vi "VFH-save_R140.vi"(7 "file path (use dialog)":path, 8 "error in (no error)":errorcluster, 10 "input":T1) -> (0 "error out":errorcluster)   [LabVIEW 2020, in "VFH-VNA_File_Handler.lvlib"]
uses:
  VFH-VNA_File_Handler.lvlib
  VFH-file_cluster-R140.ctl
  <vilib>/Utility/file.llb/Write Delimited Spreadsheet (DBL).vi
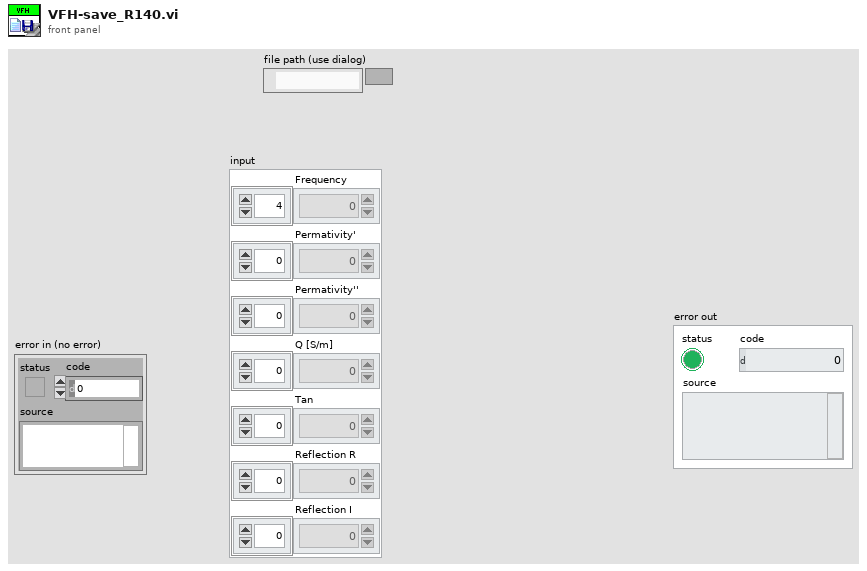
[diagram p1: front panel]
types:
  T1 = typedef "VFH-VNA_File_Handler.lvlib/VFH-file_cluster-R140.ctl" = cluster{"Frequency":dbl[], "Permativity'":dbl[], "Permativity''":dbl[], "Q [S/m]":dbl[], "Tan":dbl[], "Reflection R":dbl[], "Reflection I":dbl[]}
  T2 = enum16{"open", "replace", "create", "open or create", "replace or create", "replace or create with confirmation"}
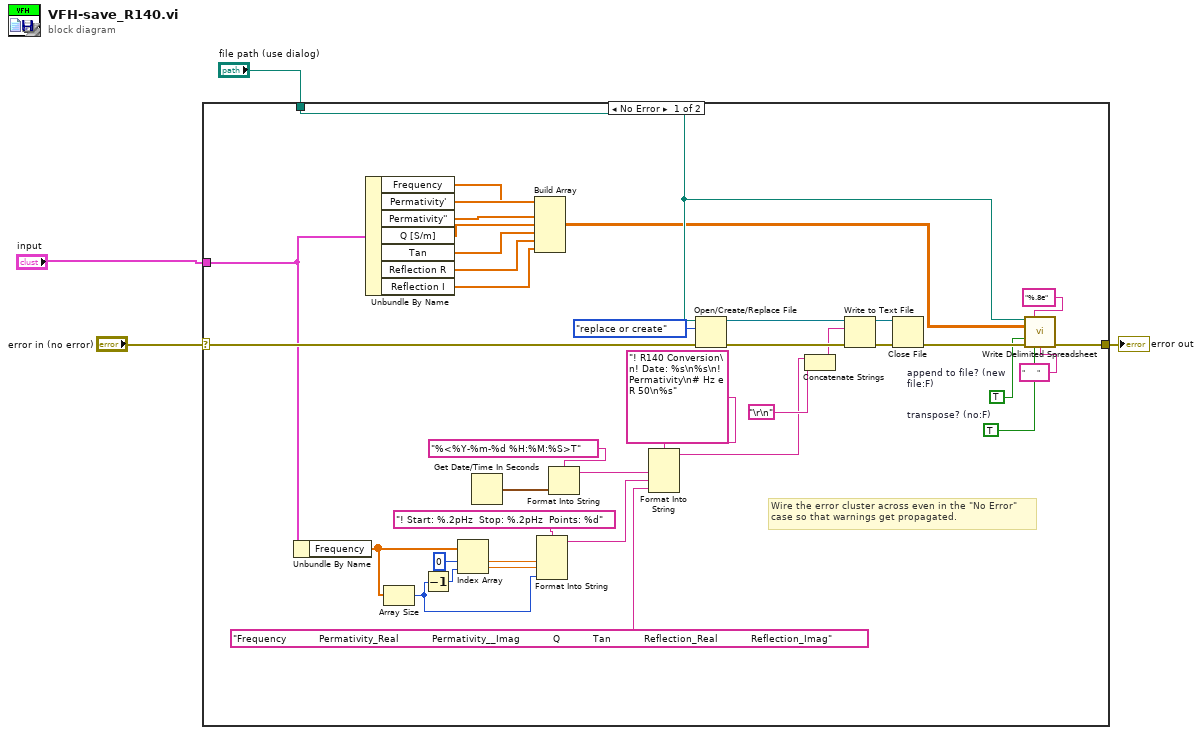
[diagram p0: block diagram]
diagram:
  n1 = case shown="No Error" "error in (no error)" {
    selector: "error in (no error)" -> [w13 w43]
    tunnel: [w5 w43] -> w1
    tunnel: "input" -> [w6 _]
    tunnel: "file path (use dialog)" -> [w22 _]
    frame No Error {
      w24 = TRUE  # append to file? (new file:F)
      w26 = TRUE  # transpose? (no:F)
      # "Wire the error cluster across even in the \"No Error\"\ncase so that warnings get propagated."
      n2 = Unbundle By Name(w6) -> ("Frequency"=w12:dbl[])
      n3 = Unbundle By Name(w6) -> ("Frequency"=w19:dbl[], "Permativity'"=w21:dbl[], "Permativity''"=w20:dbl[], "Q [S/m]"=w18:dbl[], "Tan"=w17:dbl[], "Reflection R"=w16:dbl[], "Reflection I"=w15:dbl[])
      n4 = Array Size(array=w12) -> (size(s)=w7:i32)
      n5 = Decrement(x=w7) -> (x-1=w11:i32)
      n6 = Index Array(array=w12, index #1=0 ("index"), index #2=w11) -> (element #1=w9:dbl, element #2=w8:dbl)
      n7 = Get Date/Time In Seconds() -> (seconds since 1Jan1904=w33:timestamp)
      n8 = Build Array(w19, w21, w20, w18, w17, w16, w15) -> (w14:dbl[][])
      n9 = Format Into String(format string="! Start: %.2pHz  Stop: %.2pHz  Points: %d", w9, w8, w7) -> (resulting string=w29:string)  [unwired: 2 in, 1 out]
      n10 = Format Into String(format string="%<%Y-%m-%d %H:%M:%S>T", w33) -> (resulting string=w31:string)  [unwired: 2 in, 1 out]
      n11 = Format Into String(format string="! R140 Conversion\n! Date: %s\n%s\n! Permativity\n# Hz e R 50\n%s" ("text"), w31, w29, "Frequency           Permativity_Real           Permativity__Imag           Q           Tan           Reflection_Real           Reflection_Imag" ("input 3")) -> (resulting string=w35:string)  [unwired: 2 in, 1 out]
      n12 = Open/Create/Replace File(file path (use dialog)=w22, error in=w13, operation (0:open)=T2."replace or create") -> (refnum out=w39:refnum<file>, error out=w40:errorcluster)  [unwired: 3 in, 1 out]
      n13 = Concatenate Strings(w35, "\r\n") -> (w36:string)
      n14 = Write to Text File(file (use dialog)=w39, text=w36, error in=w40) -> (refnum out=w41:refnum<file>, error out=w42:errorcluster)  [unwired: 1 in, 1 out]
      n15 = Close File(refnum=w41, error in=w42) -> (error out=w25:errorcluster)  [unwired: 1 out]
      n16 = call-poly <vilib>:"Write Delimited Spreadsheet.vi"("file path (dialog if empty)"=w22, "format (%.3f)"="%.8e", "2D data"=w14, "append to file? (new file:F)"=w24, "error in (no error)"=w25, "transpose? (no:F)"=w26, "delimiter (\\t)"="      " ("delimiter (\\t)")) -> ("error out"=w5:errorcluster)  [unwired: 7 in, 1 out]
    }
    frame Error {
    }
  }
  "error out" <- w1
